vi "实时数据时间戳 (子VI).vi"(11 "String输入":refnum<vi>) -> ()   [LabVIEW 2016, in "数据传输系统-04.lvlib"]
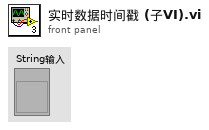
[diagram p1: front panel]
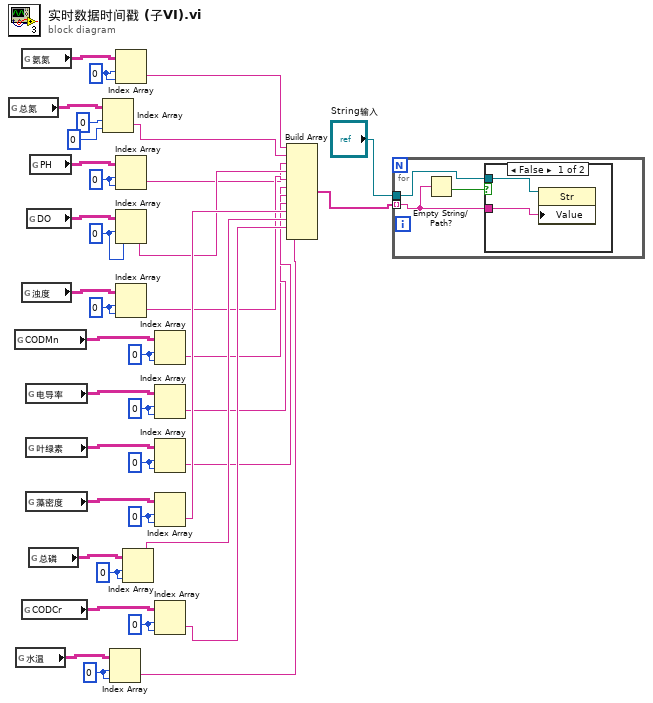
[diagram p0: block diagram]
diagram:
  w19 = 0 ("索引 (行)")
  w24 = 0 ("索引 (行)")
  w25 = 0 ("索引 (行)")
  w21 = 0 ("索引 (行)")
  w22 = 0 ("索引 (行)")
  w29 = 0 ("索引 (行)")
  w23 = 0 ("索引 (行)")
  w28 = 0 ("索引 (行)")
  w27 = 0 ("索引 (行)")
  w26 = 0 ("索引 (行)")
  w20 = 0 ("索引 (行)")
  n1 = global read "全局 所有参数.vi" "总氮"() -> (w6:string[][])
  n2 = global read "全局 所有参数.vi" "CODMn"() -> (w14:string[][])
  n3 = global read "全局 所有参数.vi" "水温"() -> (w16:string[][])
  n4 = global read "全局 所有参数.vi" "氨氮"() -> (w13:string[][])
  n5 = global read "全局 所有参数.vi" "浊度"() -> (w10:string[][])
  n6 = global read "全局 所有参数.vi" "CODCr"() -> (w15:string[][])
  n7 = global read "全局 所有参数.vi" "电导率"() -> (w9:string[][])
  n8 = global read "全局 所有参数.vi" "叶绿素"() -> (w11:string[][])
  n9 = global read "全局 所有参数.vi" "藻密度"() -> (w12:string[][])
  n10 = global read "全局 所有参数.vi" "DO"() -> (w8:string[][])
  n11 = global read "全局 所有参数.vi" "总磷"() -> (w4:string[][])
  n12 = global read "全局 所有参数.vi" "PH"() -> (w7:string[][])
  n13 = Index Array(array=w6, index (row)=0 ("索引 (行)"), index (col)=0 ("索引")) -> (element=w2:string)
  n14 = Index Array(array=w16, index (row)=w26, index (col)=w26) -> (element=w1:string)
  n15 = Index Array(array=w13, index (row)=w25, index (col)=w25) -> (element=w30:string)
  n16 = Index Array(array=w7, index (row)=w27, index (col)=w27) -> (element=w31:string)
  n17 = Index Array(array=w8, index (row)=w28, index (col)=w28) -> (element=w32:string)
  n18 = Index Array(array=w10, index (row)=w29, index (col)=w29) -> (element=w33:string)
  n19 = Index Array(array=w4, index (row)=w20, index (col)=w20) -> (element=w38:string)
  n20 = Index Array(array=w14, index (row)=w24, index (col)=w24) -> (element=w34:string)
  n21 = Index Array(array=w9, index (row)=w23, index (col)=w23) -> (element=w35:string)
  n22 = Index Array(array=w11, index (row)=w22, index (col)=w22) -> (element=w36:string)
  n23 = Index Array(array=w12, index (row)=w21, index (col)=w21) -> (element=w37:string)
  n24 = Index Array(array=w15, index (row)=w19, index (col)=w19) -> (element=w39:string)
  n25 = Build Array(w30, w2, w31, w32, w33, w34, w35, w36, w37, w38, w39, w1) -> (w17:string[])
  n26 = for {
    tunnel: w17 -> [w41] mode=indexing
    tunnel: "String输入" -> [w40]
    n27 = Empty String/Path?(string/path=w41) -> (empty?=w42:bool)
    n28 = case shown="False" w42 {
      tunnel: w41 -> [w43 _]
      tunnel: w40 -> [w44 _]
      frame False {
        n29 = property class="Str"(reference=w44, "Value"=w43) -> ()  [unwired: 1 in, 2 out]
      }
      frame True {
      }
    }
  }
